vi "Get DDG Lite Global Control Byte.vi"(11 "control":string) -> (2 "function return":u32, 3 "control out":string)   [LabVIEW 2018, in "AndorSDK.lvlib"]
doc: "EXPNETTYPE unsigned int WINAPI GetDDGLiteGlobalControlByte(unsigned char * control);"
uses:
  AndorSDK.lvlib
  ATMCD32D.dll
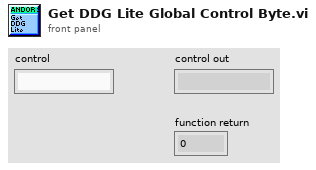
[diagram p1: front panel]
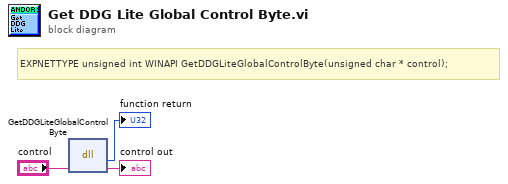
[diagram p0: block diagram]
diagram:
  # "EXPNETTYPE unsigned int WINAPI GetDDGLiteGlobalControlByte(unsigned char * control);"
  n1 = dll-call lib="PTH2babs E\nPersönliches02 - Arbeit03-HiwijobsLabviewCodelibANDOR\tAndor SDK\nATMCD32D.*" fn="GetDDGLiteGlobalControlByte"("control"="control") -> (→"function return":u32, "control"=→"control out":string)  [unwired: 3 in, 2 out]
